vi "gfitsio-open-file.vi"(8 "error in (no error)":errorcluster, 9 "read only? (T:no)":bool=TRUE, 11 "path":path) -> (0 "error out":errorcluster, 3 "gfits refnum":T1)   [LabVIEW 2019, in "gfitsio.lvlib"]
doc: "Opens an existing file for reading or writing. You cannot use this function to create or replace files."
uses:
  gfitsio.lvlib
  gfitsio-refnum.ctl
  gfitsio.dll
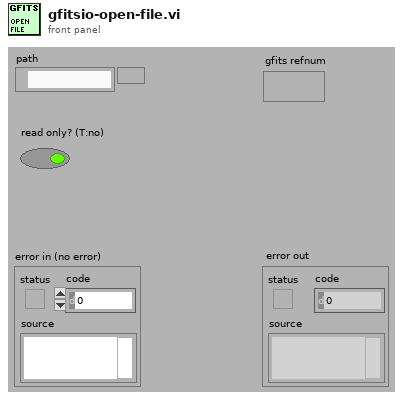
[diagram p1: front panel]
types:
  T1 = typedef "gfitsio.lvlib/gfitsio-refnum.ctl" = refnum<k1>
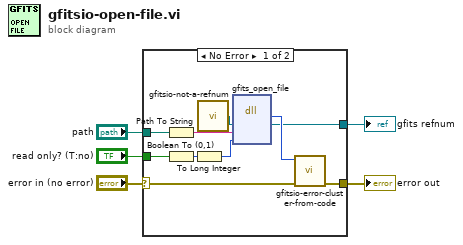
[diagram p0: block diagram]
diagram:
  n1 = case shown="No Error" "error in (no error)" {
    selector: "error in (no error)" -> [w12 w16]
    tunnel: "path" -> [w15 _]
    tunnel: [w7 _] -> w1
    tunnel: [w13 w16] -> w4
    tunnel: "read only? (T:no)" -> [w11 _]
    frame No Error {
      n2 = Path To String(path=w15) -> (string=w10:string)
      n3 = Boolean To (0,1)(Boolean=w11) -> (0, 1=w9:i16)
      n4 = To Long Integer(number=w9) -> (32bit integer=w8:i32)
      n5 = call "gfitsio-not-a-refnum.vi"() -> ("invalid gfits refnum"=w6:T1)
      n6 = dll-call lib="C:/Users/ggatling/local/GFITSIO/gfitsio/gfitsio.dll" fn="gfits_open_file"("invalid gfits refnum"=w6, "filename"=w10, "iomode"=w8) -> (w14:i32, "invalid gfits refnum"=w7:T1)  [unwired: 5 in, 2 out]
      n7 = call "gfitsio-error-cluster-from-code.vi"("error in (no error)"=w12, "error code"=w14) -> ("error out"=w13:errorcluster)  [unwired: 9 out]
    }
    frame Error {
    }
  }
  "error out" <- w4
  "gfits refnum" <- w1
